vi "Read Event Data.vi"(8 "error in (no error)":errorcluster, 11 "Variant Data":variant) -> (0 "error out":errorcluster, 2 "Event Data":variant, 3 "Event Name":string)   [LabVIEW 2011]
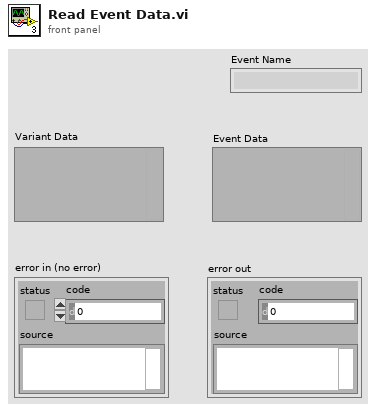
[diagram p1: front panel]
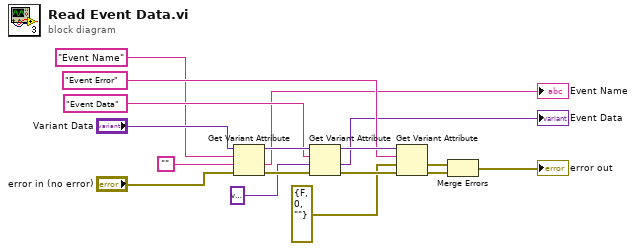
[diagram p0: block diagram]
diagram:
  n1 = Get Variant Attribute(Variant="Variant Data", name="Event Name" ("Tag"), default value (empty Variant)="", error in="error in (no error)") -> (duplicate Variant=w15:variant, value=→"Event Name":string, error out=w14:errorcluster)  [unwired: 1 out]
  n2 = Get Variant Attribute(Variant=w15, name="Event Data" ("Tag"), default value (empty Variant)=variant ("Variant"), error in=w14) -> (duplicate Variant=w12:variant, value=→"Event Data":variant, error out=w13:errorcluster)  [unwired: 1 out]
  n3 = Get Variant Attribute(Variant=w12, name="Event Error" ("Tag"), default value (empty Variant)=errorcluster {"status"=FALSE, "code"=0, "source"=""} ("error in (no error)"), error in=w13) -> (value=w4:errorcluster, error out=w6:errorcluster)  [unwired: 2 out]
  n4 = Merge Errors(w4, w6) -> (→"error out":errorcluster)
